vi "REx - NART - Commit Calibration.vi"(1 "port number(3363)":u16=3363, 2 "machine name ()":string, 11 "error in (no error)":errorcluster) -> (15 "error out":errorcluster)   [LabVIEW 2011, in "ART2 Test Panel.lvlib" / "REx - NART - Commit Calibration.lvclass"]
uses:
  REx - NART - Commit Calibration.lvclass
  LVx Folder/LVx.lvclass
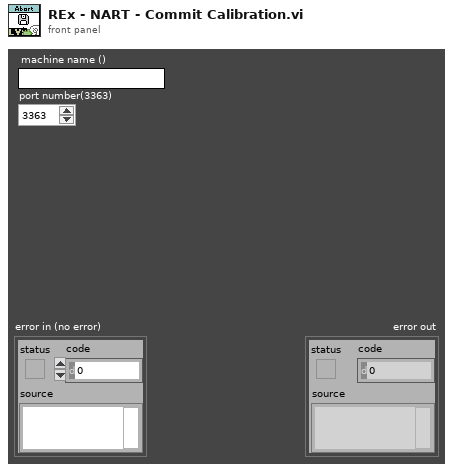
[diagram p1: front panel]
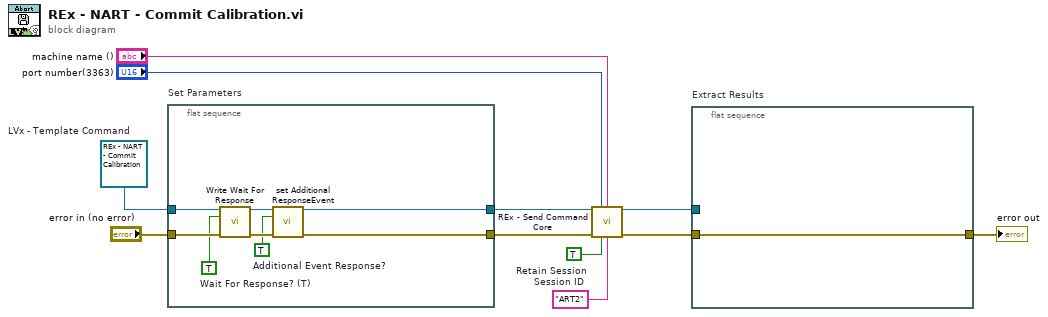
[diagram p0: block diagram]
diagram:
  w1 = "ART2"  # Session ID
  w3 = refnum<class "REx - NART - Commit Calibration.lvclass"> refnum  # LVx - Template Command
  w4 = TRUE  # Retain Session
  n1 = flat-sequence "Set Parameters" {
    tunnel: [w13] -> w11
    tunnel: "error in (no error)" -> [w16]
    tunnel: [w12] -> w8
    tunnel: w3 -> [w17]
    frame #0 {
      w14 = TRUE  # Additional Event Response?
      w15 = TRUE  # Wait For Response? (T)
      n2 = call "Write Wait For Response.vi"("LVx.lvclass in"=w17, "Wait For Response? (T)"=w15, "error in (no error)"=w16) -> ("LVx.lvclass out"=w18:refnum<class "REx - NART - Commit Calibration.lvclass">, "error out"=w19:errorcluster)  [unwired: 11 in]
      n3 = call "set Additional ResponseEvent.vi"("LVx in"=w18, "Fire Additional Event for Response?"=w14, "error in (no error)"=w19) -> ("LVx out"=w13:refnum<class "REx - NART - Commit Calibration.lvclass">, "error out"=w12:errorcluster)  [unwired: 11 in]
    }
  }
  n4 = call "REx - Send Command Core.vi"("LVx Command in"=w11, "port number(3363)"="port number(3363)", "machine name (LocalApp:\"\")"="machine name ()", "error in (no error)"=w8, "Retain Session (F)"=w4, "Session ID"=w1) -> ("LVx Command response"=w5:refnum<class "REx - NART - Commit Calibration.lvclass">, "error out"=w10:errorcluster)  [unwired: 8 in]
  n5 = flat-sequence "Extract Results" {
    tunnel: w10 -> [w20]
    tunnel: w5 -> [_]
    tunnel: [w20] -> w2
    frame #0 {
    }
  }
  "error out" <- w2
